vi "Post Test.vi"(8 "error in (no error)":errorcluster, 11 "Application in":refnum<class "Application.lvclass">) -> (0 "error out":errorcluster, 3 "Application out":refnum<class "Application.lvclass">)   [LabVIEW 2017, in "Application.lvlib" / "Application.lvclass"]
doc: "Performs any post test MES functions, if MES is enabled on the tester. The parent class implementation performs the PassLot, any child class overrides must call the parent class in addition to whatever MES calls they're doing."
uses:
  Application.lvclass
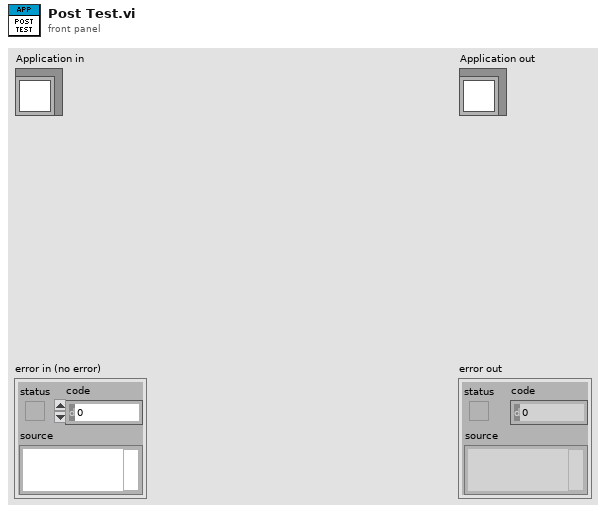
[diagram p1: front panel]
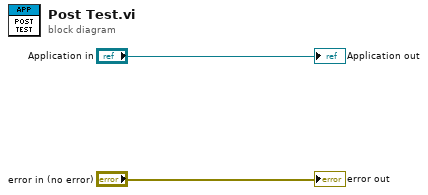
[diagram p0: block diagram]
diagram:
  "error out" <- "error in (no error)"
  "Application out" <- "Application in"
